vi "testset.vi"() -> ()   [LabVIEW 2019, in "SpectraPro.lvclass"]
uses:
  SpectraPro.lvclass
panel:
  out "Wavelength (nm) out":dbl
  out "Slit Width (um) out":dbl
  out "Grating ID":i32
  in  "VISA resource name":refnum<visa-resource-name>="COM9"
  out "error out":errorcluster
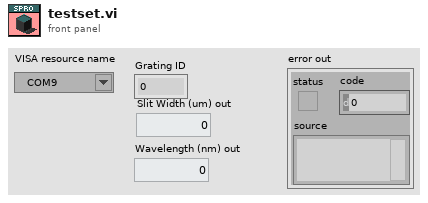
[diagram p1: front panel]
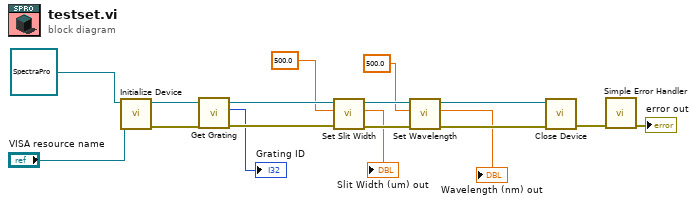
[diagram p0: block diagram]
diagram:
  n1 = call-dynamic "Initialize Device.vi"("VISA resource name"="VISA resource name", "SpectraPro in"=refnum<class "SpectraPro.lvclass"> refnum ("SpectraPro")) -> ("error out"=w16:errorcluster, "SpectraPro out"=w15:refnum<class "SpectraPro.lvclass">)  [unwired: 8 in]
  n2 = call-dynamic "Get Grating.vi"("error in (no error)"=w16, "SpectraPro in"=w15) -> ("error out"=w14:errorcluster, "Grating ID"=→"Grating ID":i32, "SpectraPro out"=w13:refnum<class "SpectraPro.lvclass">)  [unwired: 7 in]
  n3 = call-dynamic "Set Slit Width.vi"("error in (no error)"=w14, "Slit Width (um)"=500.0, "SpectraPro in"=w13) -> ("error out"=w12:errorcluster, "Slit Width (um) out"=→"Slit Width (um) out":dbl, "SpectraPro out"=w11:refnum<class "SpectraPro.lvclass">)  [unwired: 6 in]
  n4 = call-dynamic "Set Wavelength.vi"("error in (no error)"=w12, "Wavelength (nm)"=500.0, "SpectraPro in"=w11) -> ("error out"=w9:errorcluster, "Wavelength (nm) out"=→"Wavelength (nm) out":dbl, "SpectraPro out"=w10:refnum<class "SpectraPro.lvclass">)  [unwired: 6 in]
  n5 = call-dynamic "Close Device.vi"("error in (no error)"=w9, "SpectraPro in"=w10) -> ("error out"=w8:errorcluster)  [unwired: 8 in, 1 out]
  n6 = call <vilib>:"Simple Error Handler.vi"("error in (no error)"=w8) -> ("error out"=→"error out":errorcluster)  [unwired: 4 in, 4 out]
